vi "CDMA2000 On_Off.vi"(0 "VISA Resource Name":refnum<visa-resource-name>, 5 "CDMA2000 (T:ON)":bool=TRUE, 11 "error in (no error)":errorcluster {"code" format="%.0x"}) -> (4 "VISA Resource Name Out":refnum<visa-resource-name>, 15 "error out":errorcluster {"code" format="%.0x"})   [LabVIEW 2014, in "Agilent ESG Series.lvlib"]
doc: "This VI is used to enable and disable the CDMA2000 capability.\nActivating the CDMA2000 personality sets up the internal hardware to generate the currently selected CDMA2000 signal selection.\n\nThis VI is valid only on instruments E44xxB with the 101 options or on instrument E4438C with option 401."
uses:
  Agilent ESG Series.lvlib
panel:
  # "ON"
  # "OFF"
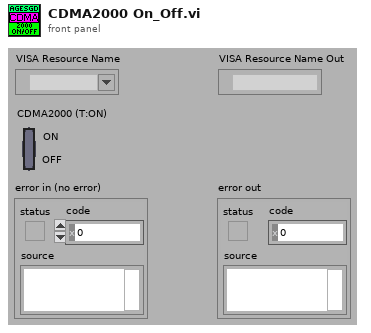
[diagram p1: front panel]
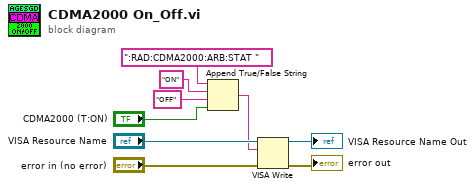
[diagram p0: block diagram]
diagram:
  n1 = Append True/False String(1:"CDMA2000 (T:ON)", 2:"OFF" ("false string"), 3:"ON" ("true string"), 4:":RAD:CDMA2000:ARB:STAT ") -> (0:w2:string)
  n2 = VISA Write(VISA resource name="VISA Resource Name", write buffer=w2, error in (no error)="error in (no error)") -> (VISA resource name out=→"VISA Resource Name Out":refnum<visa-resource-name>, error out=→"error out":errorcluster)  [unwired: 1 out]
